vi "log debug.vi"(10 "para1":cluster{}, 11 "format":string) -> (3 "function return":i32)   [LabVIEW 2019, in "apdm.lvlib"]
doc: "APDM_EXPORT int apdm_log_debug(const char *format, ...);"
uses:
  apdm.lvlib
  Lee Lab/CP FES Walking 2018/Code/Working/LabVIEW/apdm.dll
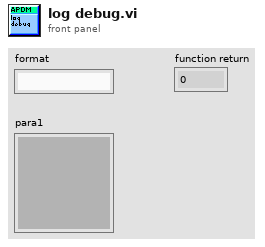
[diagram p1: front panel]
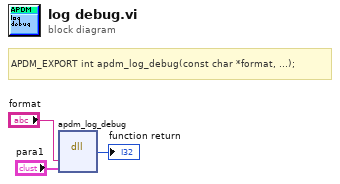
[diagram p0: block diagram]
diagram:
  # "APDM_EXPORT int apdm_log_debug(const char *format, ...);"
  n1 = dll-call lib="C:/Users/jfalesi/Dropbox/Lee Lab/CP FES Walking 2018/Code/Working/LabVIEW/apdm.*" fn="apdm_log_debug"("format"="format", "para1"="para1") -> (→"function return":i32)  [unwired: 5 in, 2 out]
